vi "Period Display Write.vi"(4 "error in (no error)":errorcluster, 5 "Value":T1, 6 "Container State":T5, 7 "Display State In":T2) -> (0 "error out":errorcluster, 3 "Display State Out":T2)   [LabVIEW 2020, in "SignalManager.xctl"]
uses:
  SignalManager.xctl
  <vilib>/_xctls/Container State.ctl
  <vilib>/_xctls/XControlSupport.lvlib
  Utility VIs/Controls/KListboxEx/Event Action.ctl
  Utility VIs/Controls/KListboxEx/KListboxEx.xctl
  Utility VIs/Controls/KListboxEx/Events.ctl
  PeriodDisplay.ctl
  State.ctl
  Events.ctl
  Event Data.ctl
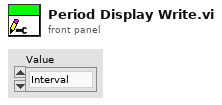
[diagram p1: front panel]
types:
  T1 = typedef "SignalManager.xctl/PeriodDisplay.ctl" = enum16{"Interval", "RepRate", "Both"}
  T2 = typedef "SignalManager.xctl/State.ctl" = cluster{"Channels":T3, "Destinations":string[], "action":string, "EventReg":refnum<event-registration>, "selectedChan":i32, "Period Display":T1, "Events":T4, "Fs (Hz)":dbl, "TDT":bool, "Frame (ms)":dbl}
  T3 = typedef "KListboxEx.xctl/Events.ctl" = cluster{"Items Changed":refnum<user-event>, "List Changed":refnum<user-event>}
  T4 = typedef "SignalManager.xctl/Events.ctl" = cluster{"Rename":refnum<user-event>}
  T5 = typedef "XControlSupport.lvlib/Container State.ctl" = cluster{"Indicator?":bool, "Run Mode?":bool, " Refnum":refnum<vi>}
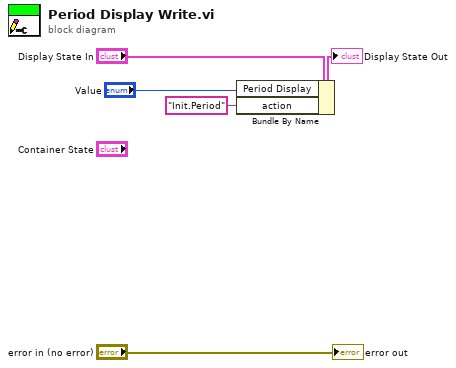
[diagram p0: block diagram]
diagram:
  n1 = Bundle By Name(cluster="Display State In", "Period Display"="Value", "action"="Init.Period") -> (→"Display State Out":T2)
  "error out" <- "error in (no error)"
